vi "TPD_Controller.vi"() -> ()   [LabVIEW 2009]
uses:
  Instance           1 22Saved   TPD_Controller .vi
  <userlib>/LV-LINK/PolySubVIs/CreateAinChan.vi
  <vilib>/addons/control/pid/pid.llb/PID (DBL).vi
  <vilib>/addons/control/pid/pid.llb/PID Gain Schedule (DBL).vi
  <userlib>/LV-LINK/PolySubVIs/OLReadSingle.vi
  <vilib>/addons/control/pid/NI_PID_pid.lvlib
  <vilib>/ptbypt/NI_PtbyPt.lvlib
panel:
  out "Pyrometer Temperature [C]":dbl format="%#_4g"
  in  "OutputPower?":bool
  in  "Resistance?":bool
  out "Resistance":dbl[](array[numeric])
  out "Measured Resistance [ohms]":dbl
  out "Gain Schedule Set?":bool
  out "Temp Schedule Set?":bool
  in  "Gain Schedule":T1(array[cluster])
  in  "Gain Schedule":bool
  out "Start Sample Temperature":dbl
  out "Temperature Setpoint [C]":dbl format="%#_5g"
  in  "Thermocouple Type":string
  out "Thermocouple Temperature":dbl[](array[numeric])
  out "Thermocouple Temperature [C]":dbl
  out "Measured Voltage [V]":dbl
  out "Measured Current [A]":dbl
  in  "Set Temperature":bool
  out "Stop Running":bool
  out "Data Points":u32
  out "Pyrometer Temperature":dbl[](array[numeric])
  out "Date":string[](array[string])
  out "Time":dbl[](array[numeric])
  out "Current Setpoint":dbl[](array[numeric])
  in  "Voltage Limit [V]":dbl min=0.0 max=20.0
  in  "Temperature Limit [C]":dbl min=-273.0 max=1300.0
  in  "Current Limit [A]":dbl min=0.0 max=14.0
  in  "Save Data":bool
  in  "Notes":string
  in  "Chamber":string
  in  "Experiment Type":string
  in  "Experimenter":string
  in  "Sample":string
  in  "Stop Heating":bool
  in  "End Program":bool
  in  "Run":bool
  in  "Reset":bool
  out "Maximum Voltage":bool
  out "Voltage":dbl[](array[numeric])
  out "Current":dbl[](array[numeric])
  out "Temperature Setpoint":dbl[](array[numeric])
  out "Maximum Current":bool
  out "Temperature and Current v. Time":T2(graph)
  out "Over Voltage":bool
  out "Over Current":bool
  out "Over Temperature":bool
  out "Start Date":string
  out "Current Setpoint [A]":dbl format="%#_3g"
  in  "Temp Schedule":cluster{"time (s)":dbl, "setpoint":dbl}[](array[cluster])
  # "TPD Controller v1.1"
  # "Experiment Setup:"
  # "Hardware Setup:"
  # "Data:"
  # "Warnings:"
  # "<14A"
  # "<20V"
  # "<1300C"
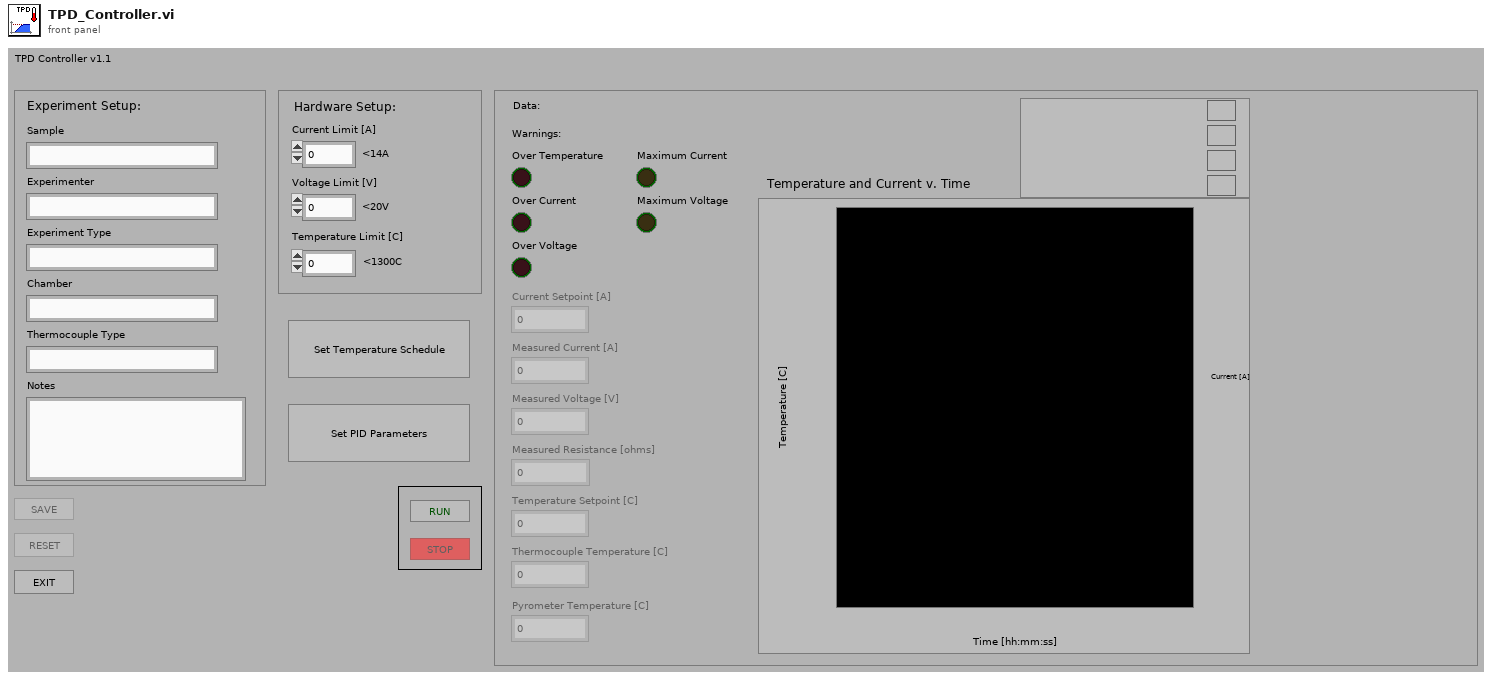
[diagram p1: front panel]
types:
  T1 = cluster{"Parameters":cluster{"Kc":dbl, "Ti":dbl, "Td":dbl}, "Maximum Temp [C]":dbl}[]
  T2 = cluster{dbl, "Temperature [C]":dbl, "setpoint":dbl, "Measured Current [A]":dbl}
  T3 = enum16{"open", "replace", "create", "open or create", "replace or create", "replace or create with confirmation"}
  T4 = cluster{"Sample":string, "Experimenter":string, "Experiment Type":string, "Chamber":string, "Thermocouple Type":string, "Notes":string}
  T5 = cluster{"proportional gain (Kc)":dbl, "integral time (Ti, min)":dbl, "derivative time (Td, min)":dbl}
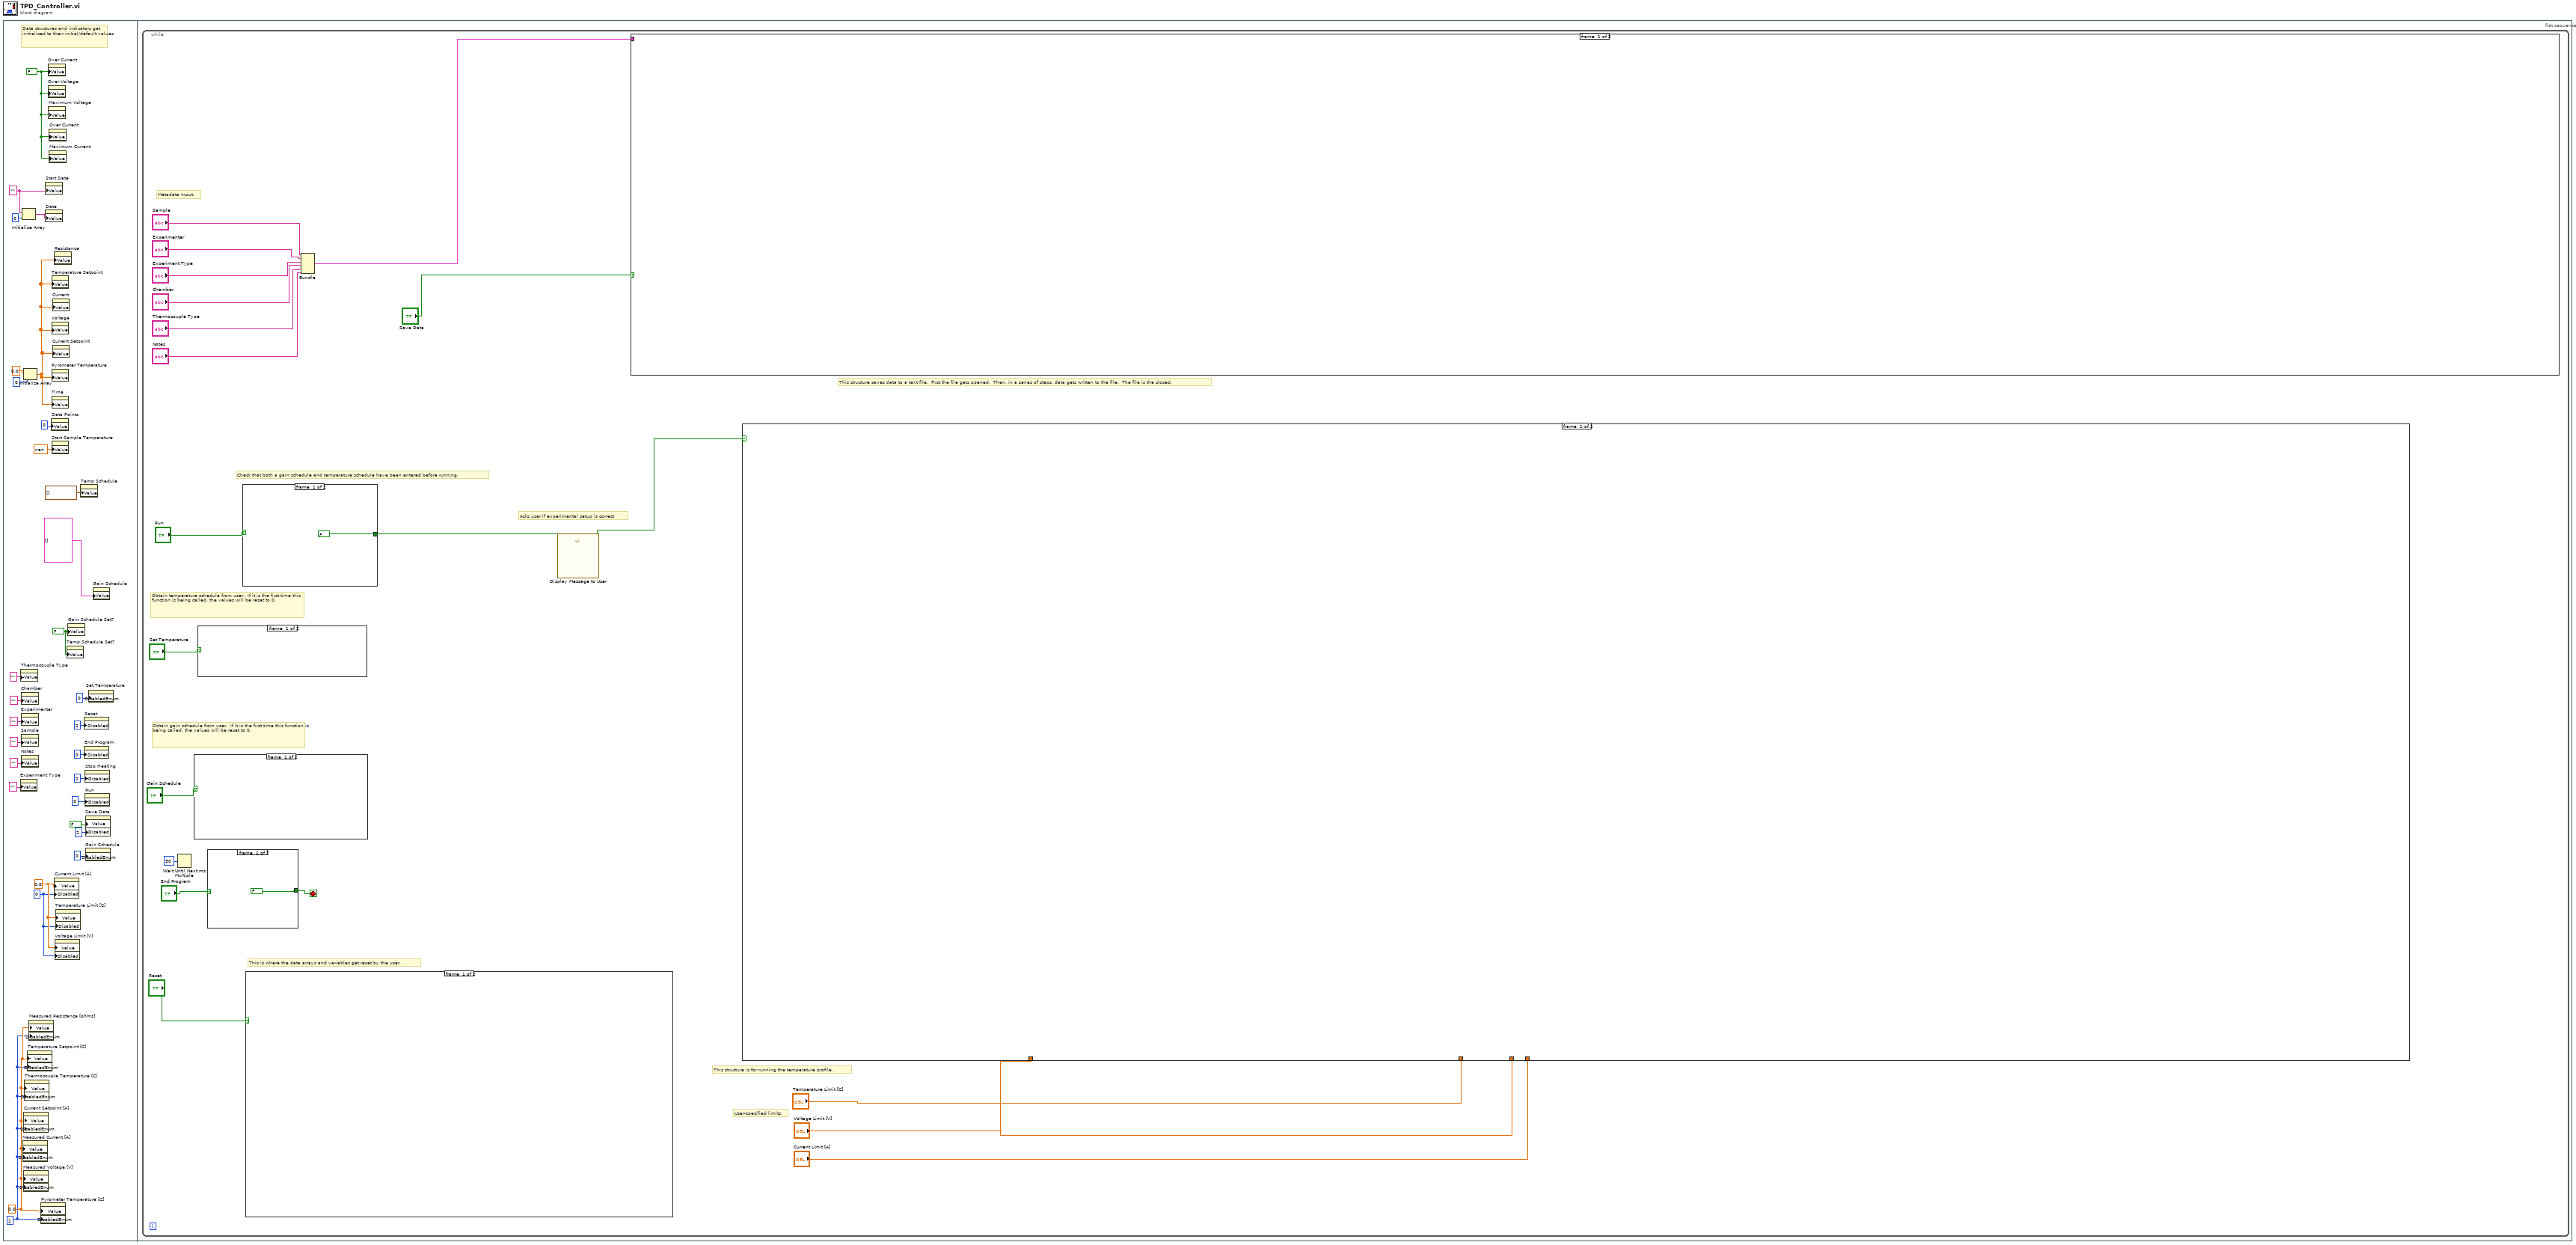
[diagram p0: block diagram]
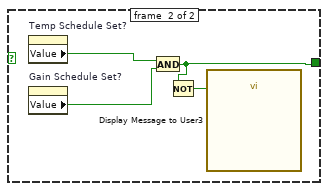
[diagram p2: hidden frame]
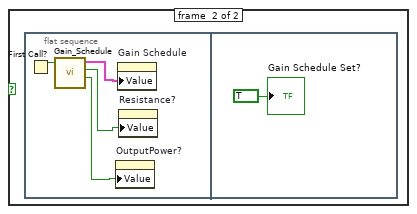
[diagram p3: hidden frame]
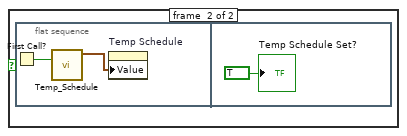
[diagram p4: hidden frame]
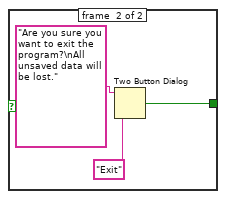
[diagram p5: hidden frame]
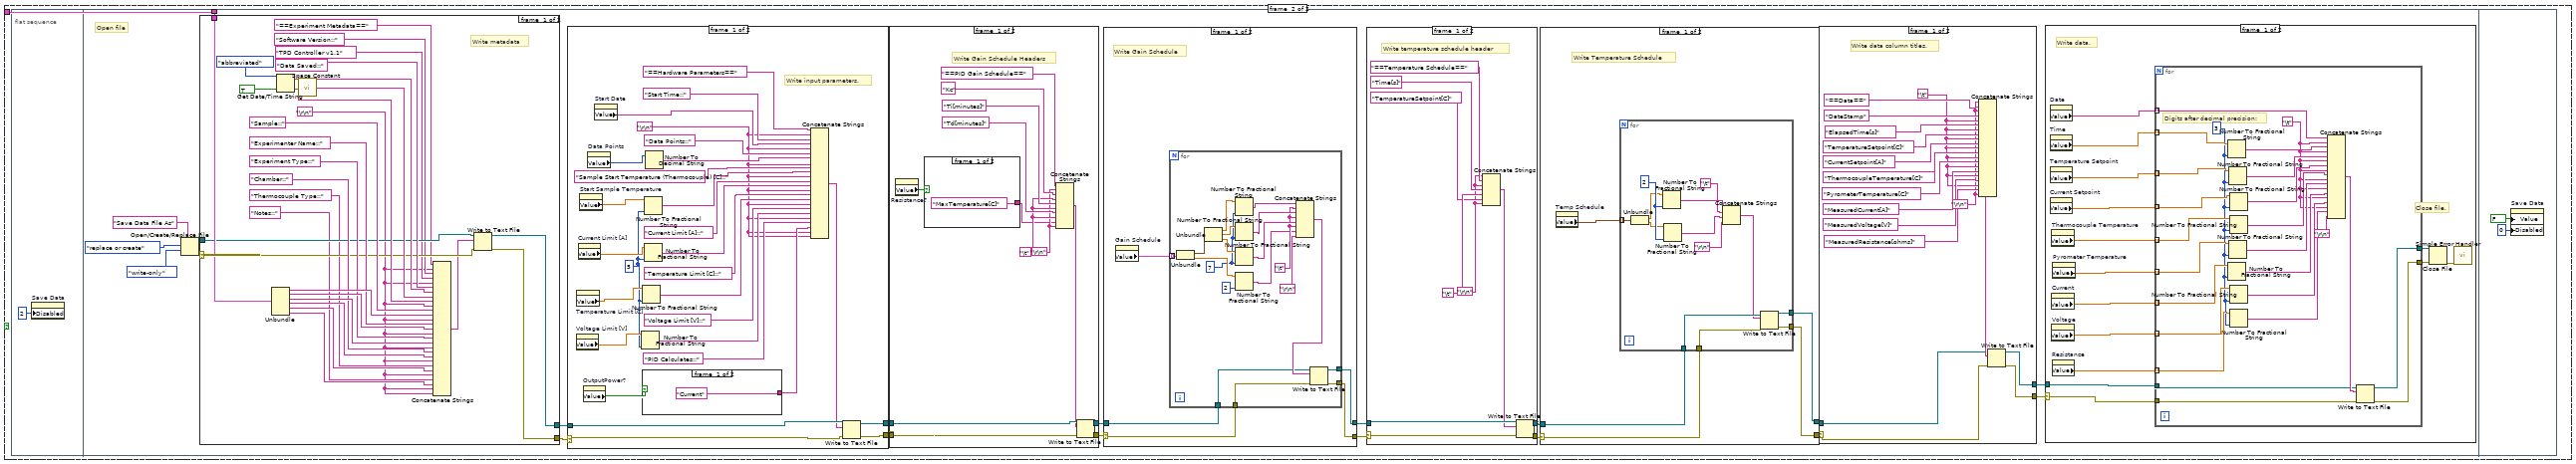
[diagram p6: hidden frame]
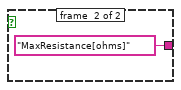
[diagram p8: hidden frame]
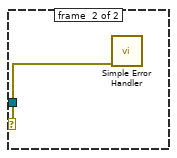
[diagram p11: hidden frame]
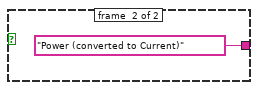
[diagram p14: hidden frame]
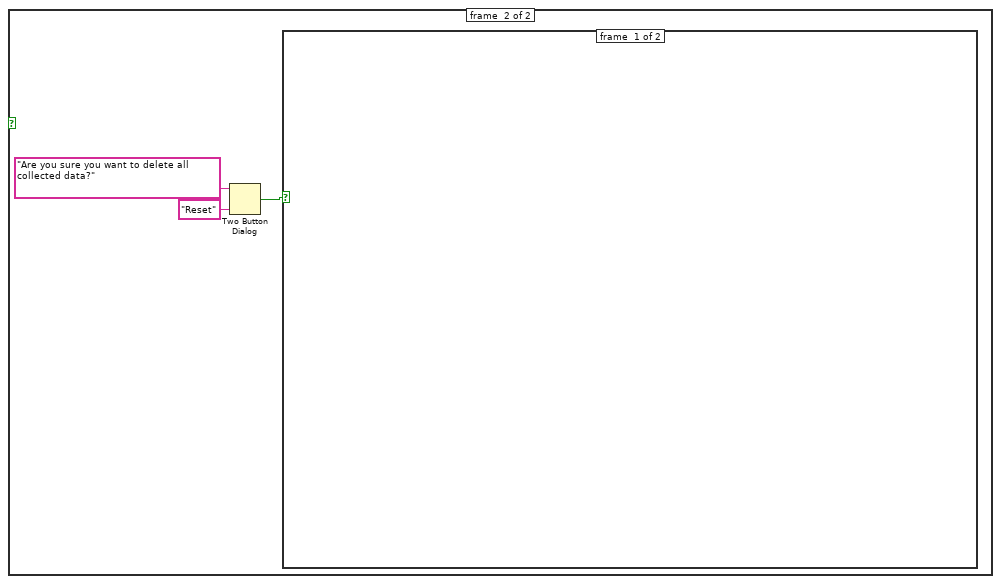
[diagram p17: hidden frame]
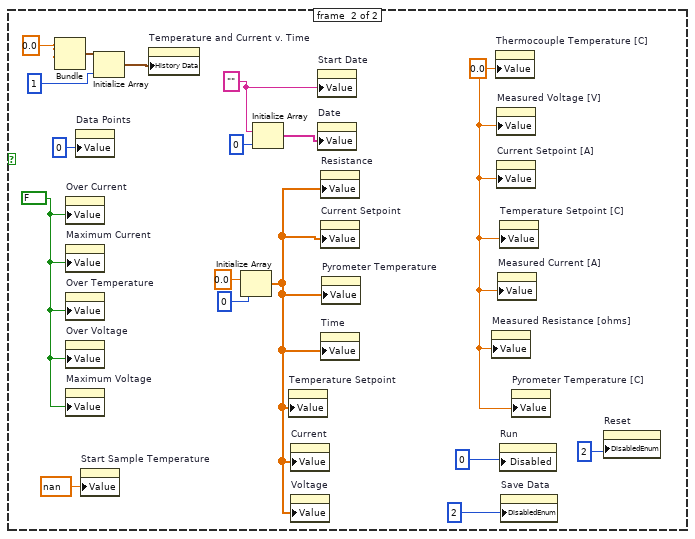
[diagram p18: hidden frame]
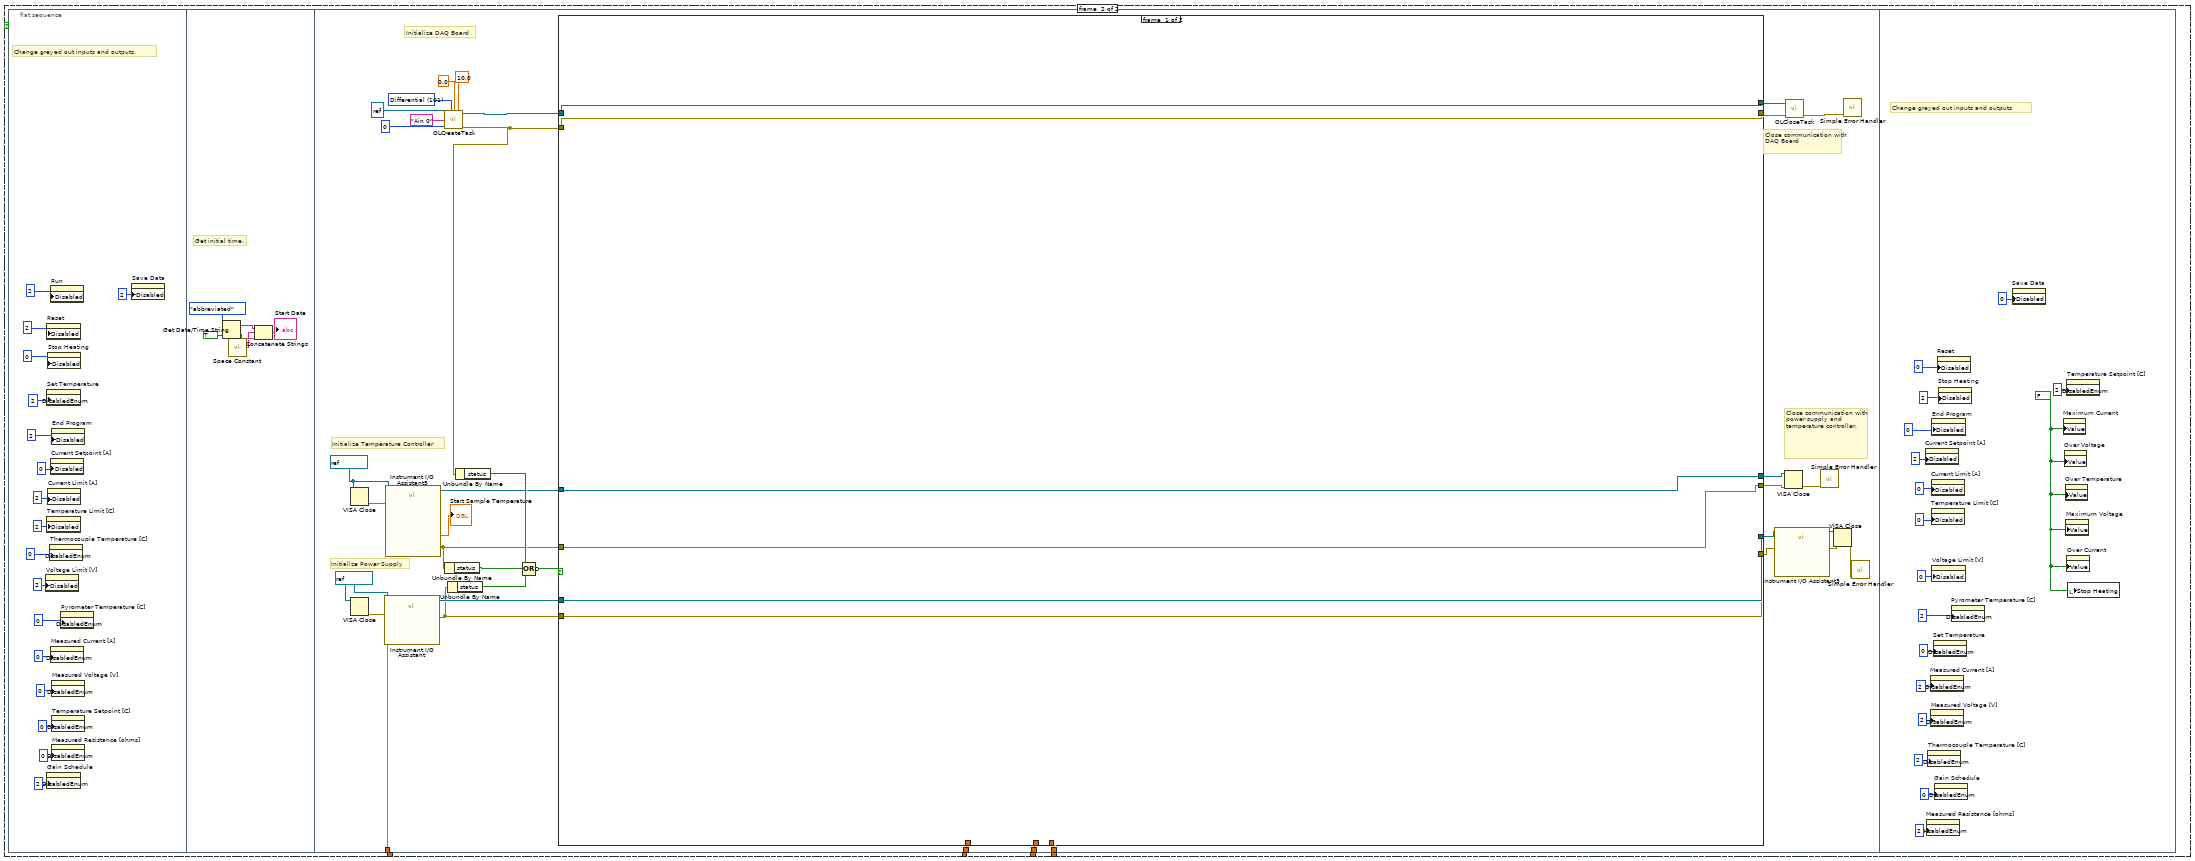
[diagram p19: hidden frame]
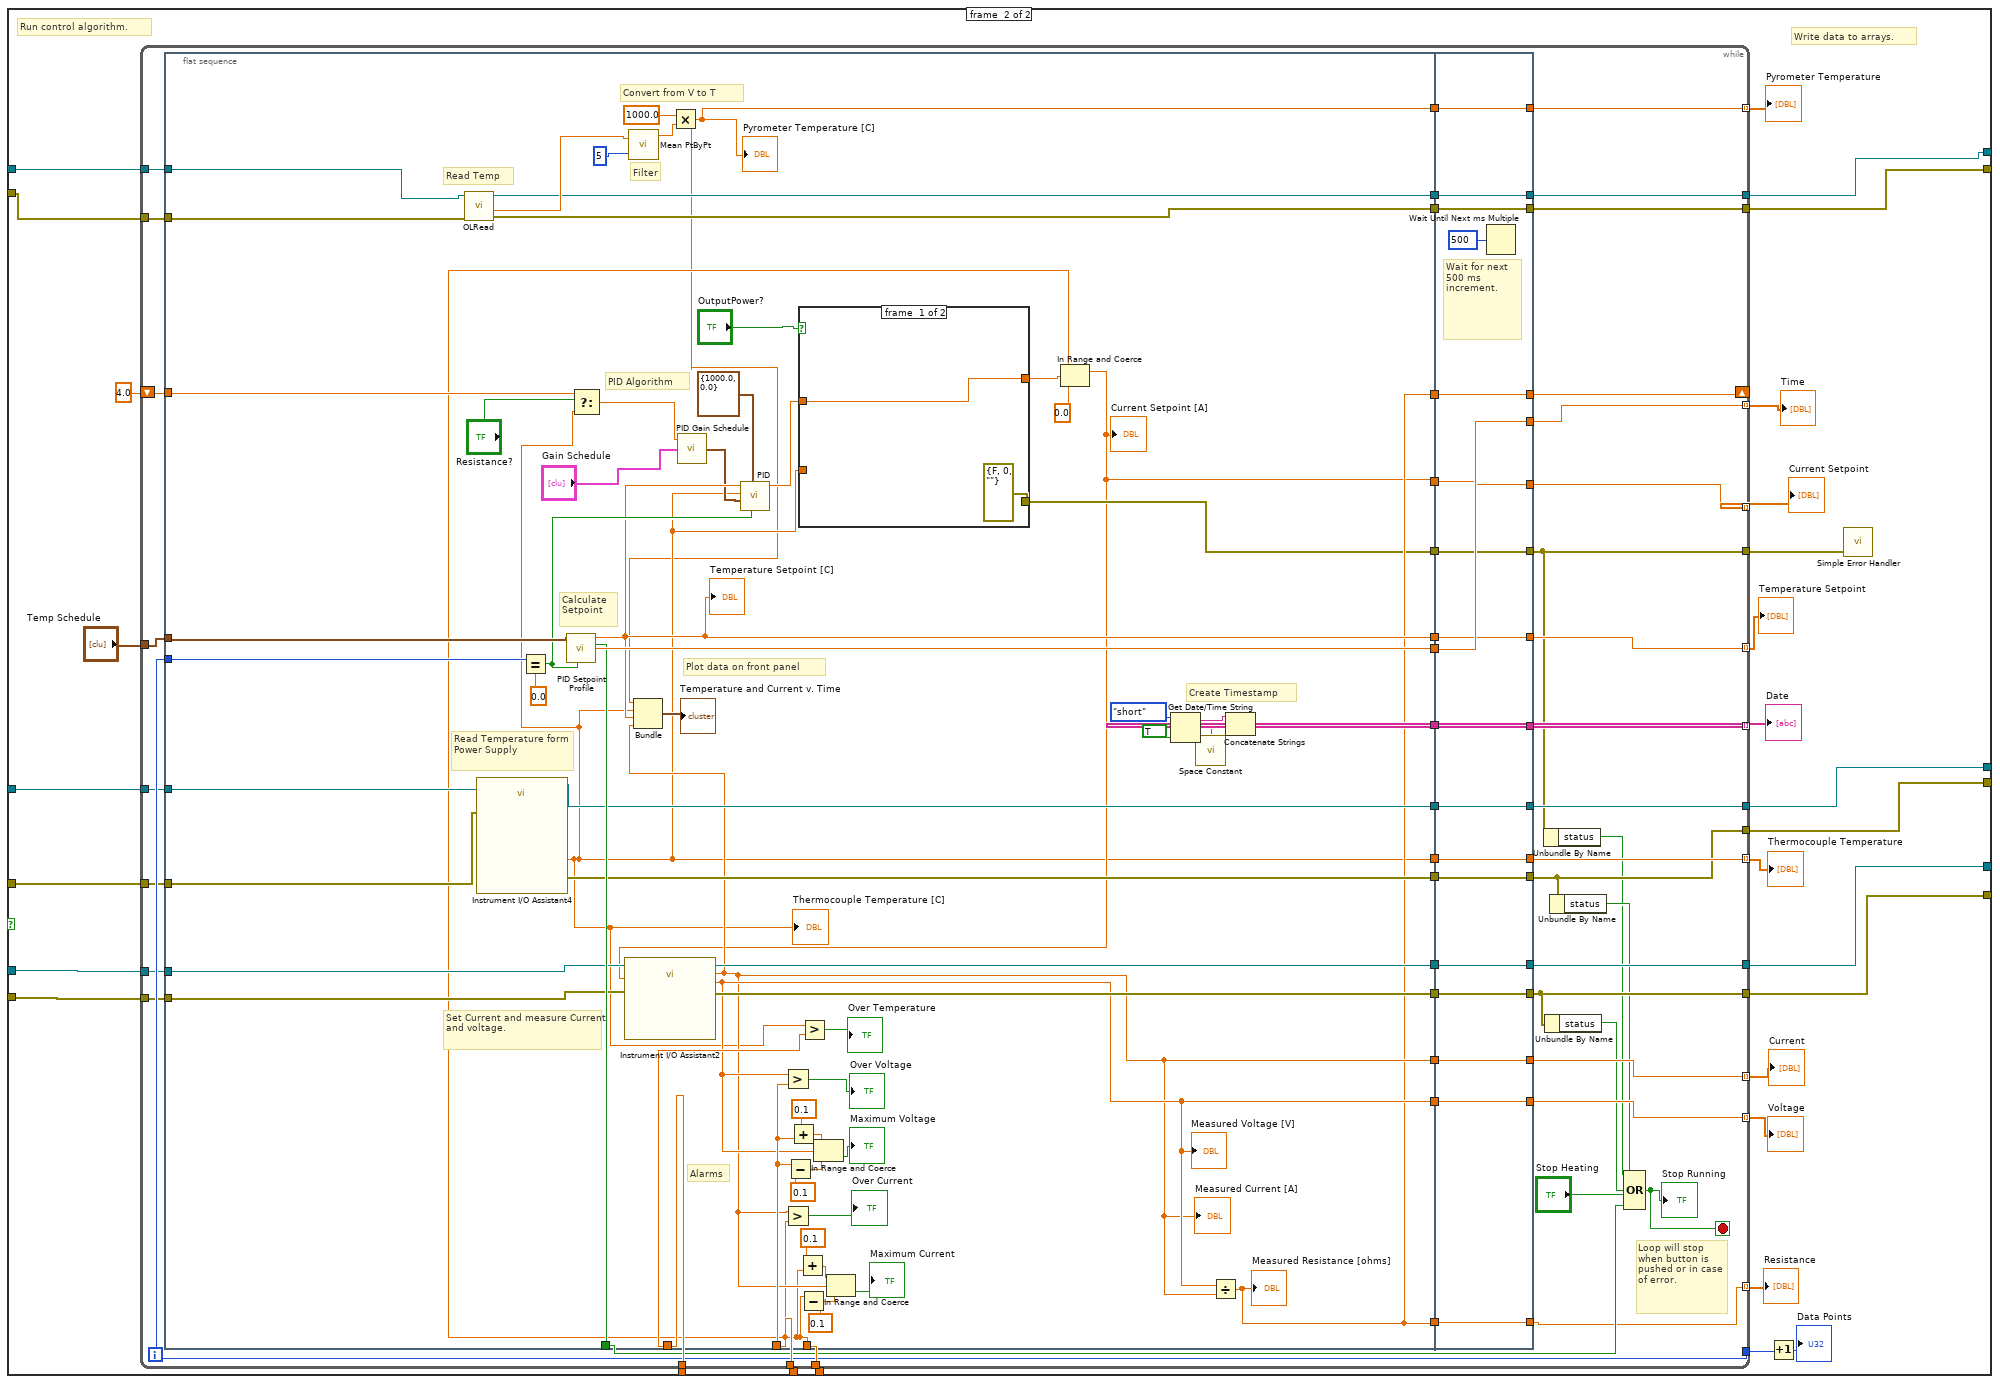
[diagram p20: hidden frame]
diagram:
  n1 = flat-sequence {
    frame #0 {
      w4 = FALSE ("Gain Schedule Set?")
      w13 = FALSE
      w11 = 0.0 ("Current Limit [A] (<11A)")
      w10 = 0
      w1 = u8 2 ("Disabled")
      w2 = 0.0 ("Current Temperature [C]")
      w23 = "" ("Start Date")
      # "Data structures and indicators get initialized to their initial/default values."
      n2 = property on="Experiment Type" class="Str"("Value"="" ("Experiment Type")) -> ()  [unwired: 2 in, 2 out]
      n3 = property on="Thermocouple Type" class="Str"("Value"="" ("Chamber")) -> ()  [unwired: 2 in, 2 out]
      n4 = property on="Chamber" class="Str"("Value"="" ("Chamber")) -> ()  [unwired: 2 in, 2 out]
      n5 = property on="Experimenter" class="Str"("Value"="" ("Experimenter")) -> ()  [unwired: 2 in, 2 out]
      n6 = property on="Sample" class="Str"("Value"="" ("Sample")) -> ()  [unwired: 2 in, 2 out]
      n7 = property on="Notes" class="Str"("Value"="" ("Notes")) -> ()  [unwired: 2 in, 2 out]
      n8 = Initialize Array(w23, 0 ("dimension size")) -> (w24:string[])
      n9 = property on="Measured Current [A]" class="DigNum (strict)"("Value"=w2, "DisabledEnum"=w1) -> ()  [unwired: 2 in, 2 out]
      n10 = Initialize Array(0.0 ("element"), 0 ("dimension size")) -> (w3:dbl[])
      n11 = property on="Measured Voltage [V]" class="DigNum (strict)"("Value"=w2, "DisabledEnum"=w1) -> ()  [unwired: 2 in, 2 out]
      n12 = property on="Current Setpoint [A]" class="DigNum (strict)"("Value"=w2, "DisabledEnum"=w1) -> ()  [unwired: 2 in, 2 out]
      n13 = property on="Thermocouple Temperature [C]" class="DigNum (strict)"("Value"=w2, "DisabledEnum"=w1) -> ()  [unwired: 2 in, 2 out]
      n14 = property on="Temperature Setpoint [C]" class="DigNum (strict)"("Value"=w2, "DisabledEnum"=w1) -> ()  [unwired: 2 in, 2 out]
      n15 = property on="Measured Resistance [ohms]" class="DigNum (strict)"("Value"=w2, "DisabledEnum"=w1) -> ()  [unwired: 2 in, 2 out]
      n16 = property on="Pyrometer Temperature [C]" class="DigNum (strict)"("Value"=w2, "DisabledEnum"=w1) -> ()  [unwired: 2 in, 2 out]
      n17 = property on="Start Date" class="Str"("Value"=w23) -> ()  [unwired: 2 in, 2 out]
      n18 = property on="Date" class="Arr (strict)"("Value"=w24) -> ()  [unwired: 2 in, 2 out]
      n19 = property on="Over Current" class="Bool (strict)"("Value"=w13) -> ()  [unwired: 2 in, 2 out]
      n20 = property on="Over Voltage" class="Bool (strict)"("Value"=w13) -> ()  [unwired: 2 in, 2 out]
      n21 = property on="Maximum Voltage" class="Bool (strict)"("Value"=w13) -> ()  [unwired: 2 in, 2 out]
      n22 = property on="Over Current" class="Bool (strict)"("Value"=w13) -> ()  [unwired: 2 in, 2 out]
      n23 = property on="Maximum Current" class="Bool (strict)"("Value"=w13) -> ()  [unwired: 2 in, 2 out]
      n24 = property on="Data Points" class="DigNum (strict)"("Value"=u32 0 ("Data Points")) -> ()  [unwired: 2 in, 2 out]
      n25 = property on="Temperature Setpoint" class="Arr (strict)"("Value"=w3) -> ()  [unwired: 2 in, 2 out]
      n26 = property on="Voltage" class="Arr (strict)"("Value"=w3) -> ()  [unwired: 2 in, 2 out]
      n27 = property on="Pyrometer Temperature" class="Arr (strict)"("Value"=w3) -> ()  [unwired: 2 in, 2 out]
      n28 = property on="Time" class="Arr (strict)"("Value"=w3) -> ()  [unwired: 2 in, 2 out]
      n29 = property on="Start Sample Temperature" class="DigNum (strict)"("Value"=nan ("Start Sample Temperature")) -> ()  [unwired: 2 in, 2 out]
      n30 = property on="Current" class="Arr (strict)"("Value"=w3) -> ()  [unwired: 2 in, 2 out]
      n31 = property on="Current Setpoint" class="Arr (strict)"("Value"=w3) -> ()  [unwired: 2 in, 2 out]
      n32 = property on="Resistance" class="Arr (strict)"("Value"=w3) -> ()  [unwired: 2 in, 2 out]
      n33 = property on="Current Limit [A]" class="DigNum (strict)"("Value"=w11, "Disabled"=w10) -> ()  [unwired: 2 in, 2 out]
      n34 = property on="Voltage Limit [V]" class="DigNum (strict)"("Value"=w11, "Disabled"=w10) -> ()  [unwired: 2 in, 2 out]
      n35 = property on="Temperature Limit [C]" class="DigNum (strict)"("Value"=w11, "Disabled"=w10) -> ()  [unwired: 2 in, 2 out]
      n36 = property on="Temp Schedule Set?" class="Bool (strict)"("Value"=w4) -> ()  [unwired: 2 in, 2 out]
      n37 = property on="Gain Schedule Set?" class="Bool (strict)"("Value"=w4) -> ()  [unwired: 2 in, 2 out]
      n38 = property on="Temp Schedule" class="Arr (strict)"("Value"=cluster{"time (s)":dbl, "setpoint":dbl}[] [] ("Temp Schedule")) -> ()  [unwired: 2 in, 2 out]
      n39 = property on="Reset" class="Bool"("Disabled"=u8 2) -> ()  [unwired: 2 in, 2 out]
      n40 = property on="End Program" class="Bool"("Disabled"=u8 0) -> ()  [unwired: 2 in, 2 out]
      n41 = property on="Stop Heating" class="Bool (strict)"("Disabled"=u8 2) -> ()  [unwired: 2 in, 2 out]
      n42 = property on="Run" class="Bool"("Disabled"=u8 0) -> ()  [unwired: 2 in, 2 out]
      n43 = property on="Save Data" class="Bool (strict)"("Value"=FALSE, "Disabled"=u8 2) -> ()  [unwired: 2 in, 2 out]
      n44 = property on="Gain Schedule" class="Bool"("DisabledEnum"=u8 0 ("Disabled")) -> ()  [unwired: 2 in, 2 out]
      n45 = property on="Set Temperature" class="Bool"("DisabledEnum"=0) -> ()  [unwired: 2 in, 2 out]
      n46 = property on="Gain Schedule" class="Arr (strict)"("Value"=T1 [] ("Gain Schedule 2")) -> ()  [unwired: 2 in, 2 out]
    }
    frame #1 {
      n47 = while {
        stop <- w42 stop-if-true
        # "Obtain gain schedule from user.  If it is the first time this function is being called, the values will be reset to 0."
        # "Check that both a gain schedule and temperature schedule have been entered before running."
        # "Obtain temperature schedule from user.  If it is the first time this function is being called, the values will be reset to 0."
        # "Asks user if experimental setup is correct"
        # "User-specified limits:"
        # "Metadata Input:"
        # "This structure saves data to a text file.  First the file gets opened.  Then, in a series of steps, data gets written to the file.  The file is the closed."
        # "This is where the data arrays and variables get reset by the user."
        # "This structure is for running the temperature profile."
        n48 = Wait Until Next ms Multiple(millisecond multiple=u32 50) -> ()  [unwired: 1 out]
        n49 = case shown="True" "Gain Schedule" {
          frame #0 {
          }
          frame #1 {
            n50 = flat-sequence {
              frame #0 {
                n51 = First Call?() -> (First Call?: T/F=w59:bool)
                n52 = call "Gain_Schedule.vi"("Initialize?"=w59) -> ("Outpower?"=w56:bool, "Resistance?"=w57:bool, "Array 2"=w58:T1)  [unwired: 8 in]
                n53 = property on="OutputPower?" class="Bool (strict)"("Value"=w56) -> ()  [unwired: 2 in, 2 out]
                n54 = property on="Gain Schedule" class="Arr (strict)"("Value"=w58) -> ()  [unwired: 2 in, 2 out]
                n55 = property on="Resistance?" class="Bool (strict)"("Value"=w57) -> ()  [unwired: 2 in, 2 out]
              }
              frame #1 {
                "Gain Schedule Set?" <- TRUE ("Gain Schedule Set?")
              }
            }
          }
        }
        n56 = case shown="True" "Set Temperature" {
          frame #0 {
          }
          frame #1 {
            n57 = flat-sequence {
              frame #0 {
                n58 = First Call?() -> (First Call?: T/F=w62:bool)
                n59 = call "Temp_Schedule.vi"("Initialize?"=w62) -> (3:w61:cluster{"time (s)":dbl, "setpoint":dbl}[])  [unwired: 9 in]
                n60 = property on="Temp Schedule" class="Arr (strict)"("Value"=w61) -> ()  [unwired: 2 in, 2 out]
              }
              frame #1 {
                "Temp Schedule Set?" <- TRUE ("Temp Schedule Set?")
              }
            }
          }
        }
        n61 = case shown="True" "End Program" {
          tunnel: [FALSE w65] -> w42
          frame #0 {
          }
          frame #1 {
            n62 = Two Button Dialog(message="Are you sure you want to exit the program?\nAll unsaved data will be lost.", 2:"Exit" ("T button name (\"OK\")")) -> (T button?=w65:bool)  [unwired: 1 in]
          }
        }
        n63 = case shown="True" "Run" {
          tunnel: [FALSE w53] -> w31
          frame #0 {
          }
          frame #1 {
            n64 = property on="Temp Schedule Set?" class="Bool (strict)"() -> ("Value"=w55:bool)  [unwired: 2 in, 2 out]
            n65 = property on="Gain Schedule Set?" class="Bool (strict)"() -> ("Value"=w54:bool)  [unwired: 2 in, 2 out]
            n66 = And(x=w55, y=w54) -> (x .and. y?=w53:bool)
            n67 = Not(x=w53) -> (.not. x?=w52:bool)
            n68 = call "Display Message to User3"("Enable"=w52) -> ()  [unwired: 9 in, 2 out]
          }
        }
        n69 = case shown="True" "Reset" {
          frame #0 {
          }
          frame #1 {
            n70 = Two Button Dialog(message="Are you sure you want to delete all collected data?", 2:"Reset" ("T button name (\"OK\")")) -> (T button?=w290:bool)  [unwired: 1 in]
            n71 = case shown="True" w290 {
              frame #0 {
              }
              frame #1 {
                w292 = 0.0 ("Thermocouple Temperature [C]")
                w298 = FALSE
                w291 = 0.0
                w307 = "" ("Start Date")
                n72 = Bundle(w291, w291, w291, w291) -> (w300:cluster{dbl, dbl, dbl, dbl})  [unwired: 1 in]
                n73 = property on="Over Current" class="Bool (strict)"("Value"=w298) -> ()  [unwired: 2 in, 2 out]
                n74 = property on="Maximum Current" class="Bool (strict)"("Value"=w298) -> ()  [unwired: 2 in, 2 out]
                n75 = property on="Over Temperature" class="Bool (strict)"("Value"=w298) -> ()  [unwired: 2 in, 2 out]
                n76 = property on="Over Voltage" class="Bool (strict)"("Value"=w298) -> ()  [unwired: 2 in, 2 out]
                n77 = property on="Maximum Voltage" class="Bool (strict)"("Value"=w298) -> ()  [unwired: 2 in, 2 out]
                n78 = property on="Data Points" class="DigNum (strict)"("Value"=u32 0 ("Data Points")) -> ()  [unwired: 2 in, 2 out]
                n79 = property on="Start Sample Temperature" class="DigNum (strict)"("Value"=nan ("Start Sample Temperature")) -> ()  [unwired: 2 in, 2 out]
                n80 = Initialize Array(w300, 1 ("dimension size")) -> (w299:cluster{dbl, dbl, dbl, dbl}[])
                n81 = property on="Temperature and Current v. Time" class="WFChart (strict)"("History Data"=w299) -> ()  [unwired: 2 in, 2 out]
                n82 = Initialize Array(0.0 ("element"), 0 ("dimension size")) -> (w295:dbl[])
                n83 = Initialize Array(w307, 0 ("dimension size")) -> (w305:string[])
                n84 = property on="Temperature Setpoint" class="Arr (strict)"("Value"=w295) -> ()  [unwired: 2 in, 2 out]
                n85 = property on="Current" class="Arr (strict)"("Value"=w295) -> ()  [unwired: 2 in, 2 out]
                n86 = property on="Voltage" class="Arr (strict)"("Value"=w295) -> ()  [unwired: 2 in, 2 out]
                n87 = property on="Start Date" class="Str"("Value"=w307) -> ()  [unwired: 2 in, 2 out]
                n88 = property on="Date" class="Arr (strict)"("Value"=w305) -> ()  [unwired: 2 in, 2 out]
                n89 = property on="Resistance" class="Arr (strict)"("Value"=w295) -> ()  [unwired: 2 in, 2 out]
                n90 = property on="Current Setpoint" class="Arr (strict)"("Value"=w295) -> ()  [unwired: 2 in, 2 out]
                n91 = property on="Time" class="Arr (strict)"("Value"=w295) -> ()  [unwired: 2 in, 2 out]
                n92 = property on="Pyrometer Temperature" class="Arr (strict)"("Value"=w295) -> ()  [unwired: 2 in, 2 out]
                n93 = property on="Measured Resistance [ohms]" class="DigNum (strict)"("Value"=w292) -> ()  [unwired: 2 in, 2 out]
                n94 = property on="Thermocouple Temperature [C]" class="DigNum (strict)"("Value"=w292) -> ()  [unwired: 2 in, 2 out]
                n95 = property on="Measured Voltage [V]" class="DigNum (strict)"("Value"=w292) -> ()  [unwired: 2 in, 2 out]
                n96 = property on="Current Setpoint [A]" class="DigNum (strict)"("Value"=w292) -> ()  [unwired: 2 in, 2 out]
                n97 = property on="Measured Current [A]" class="DigNum (strict)"("Value"=w292) -> ()  [unwired: 2 in, 2 out]
                n98 = property on="Temperature Setpoint [C]" class="DigNum (strict)"("Value"=w292) -> ()  [unwired: 2 in, 2 out]
                n99 = property on="Run" class="Bool"("Disabled"=0) -> ()  [unwired: 2 in, 2 out]
                n100 = property on="Save Data" class="Bool (strict)"("DisabledEnum"=2 ("Disabled")) -> ()  [unwired: 2 in, 2 out]
                n101 = property on="Pyrometer Temperature [C]" class="DigNum (strict)"("Value"=w292) -> ()  [unwired: 2 in, 2 out]
                n102 = property on="Reset" class="Bool"("DisabledEnum"=2 ("Disabled")) -> ()  [unwired: 2 in, 2 out]
              }
            }
          }
        }
        n103 = Bundle("Sample"="Sample", "Experimenter"="Experimenter", "Experiment Type"="Experiment Type", "Chamber"="Chamber", "Thermocouple Type"="Thermocouple Type", "Notes"="Notes") -> (w44:T4)  [unwired: 1 in]
        n104 = call "Display Message to User"("Enable"=w31) -> ("Yes"=w39:bool)  [unwired: 9 in, 1 out]
        n105 = case shown="True" "Save Data" {
          tunnel: w44 -> [_ w68]
          frame #0 {
          }
          frame #1 {
            n106 = flat-sequence {
              tunnel: w68 -> [w85]
              frame #0 {
                n107 = property on="Save Data" class="Bool (strict)"("Disabled"=u8 2) -> ()  [unwired: 2 in, 2 out]
              }
              frame #1 {
                # "Open file"
                n108 = Open/Create/Replace File(prompt="Save Data File As", operation (0:open)=T3."replace or create", access (0:read/write)=enum16{"read/write", "read-only", "write-only"}."write-only") -> (refnum out=w84:refnum<file>, error out=w86:errorcluster)  [unwired: 3 in, 1 out]
                n109 = case shown="No Error" w86 {
                  selector: w86 -> [w269 w285]
                  tunnel: w85 -> [w283 _]
                  tunnel: w84 -> [w267 w284]
                  tunnel: [w266 w285] -> w83
                  tunnel: [w265 w284] -> w82
                  frame #0 {
                    w256 = "\r\n"
                    # "Write metadata"
                    n110 = Unbundle(w283) -> ("Sample"=w277:string, "Experimenter"=w275:string, "Experiment Type"=w273:string, "Chamber"=w271:string, "Thermocouple Type"=w270:string, "Notes"=w258:string)
                    n111 = Get Date/Time String(date format (0)=enum16{"short", "long", "abbreviated"}."abbreviated", want seconds? (F)=TRUE) -> (date string=w281:string, time string=w279:string)  [unwired: 1 in]
                    n112 = call <vilib>:"Space Constant.vi"() -> ("String"=w280:string)
                    n113 = Concatenate Strings("==Experiment Metadata==", w256, "Software Version::", "TPD Controller v1.1", w256, "Data Saved::", w281, w280, w279, w256, "Sample::", w277, w256, "Experimenter Name::", w275, w256, "Experiment Type::", w273, w256, "Chamber::", w271, w256, "Thermocouple Type::", w270, w256, "Notes::", w258, w256, w256) -> (w268:string)
                    n114 = Write to Text File(file (use dialog)=w267, text=w268, error in=w269) -> (refnum out=w265:refnum<file>, error out=w266:errorcluster)  [unwired: 1 in, 1 out]
                  }
                  frame #1 {
                  }
                }
                n115 = case shown="No Error" w83 {
                  selector: w83 -> [w243 w255]
                  tunnel: w82 -> [w244 w254]
                  tunnel: [w238 w255] -> w74
                  tunnel: [w237 w254] -> w75
                  frame #0 {
                    w229 = i16 5 ("precision (6)")
                    w224 = "\r\n"
                    # "Write input parameters."
                    n116 = property on="Voltage Limit [V]" class="DigNum (strict)"() -> ("Value"=w239:dbl)  [unwired: 2 in, 2 out]
                    n117 = property on="Temperature Limit [C]" class="DigNum (strict)"() -> ("Value"=w240:dbl)  [unwired: 2 in, 2 out]
                    n118 = property on="Current Limit [A]" class="DigNum (strict)"() -> ("Value"=w241:dbl)  [unwired: 2 in, 2 out]
                    n119 = property on="Start Sample Temperature" class="DigNum (strict)"() -> ("Value"=w232:dbl)  [unwired: 2 in, 2 out]
                    n120 = property on="OutputPower?" class="Bool (strict)"() -> ("Value"=w226:bool)  [unwired: 2 in, 2 out]
                    n121 = property on="Data Points" class="DigNum (strict)"() -> ("Value"=w235:u32)  [unwired: 2 in, 2 out]
                    n122 = property on="Start Date" class="Str"() -> ("Value"=w236:string)  [unwired: 2 in, 2 out]
                    n123 = Number To Fractional String(number=w239, precision (6)=w229) -> (F-format string=w233:string)  [unwired: 2 in]
                    n124 = Number To Fractional String(number=w240, precision (6)=w229) -> (F-format string=w245:string)  [unwired: 2 in]
                    n125 = case shown="True" w226 {
                      tunnel: ["Current" "Power (converted to Current)"] -> w225
                      frame #0 {
                      }
                      frame #1 {
                      }
                    }
                    n126 = Number To Fractional String(number=w232, precision (6)=w229) -> (F-format string=w231:string)  [unwired: 2 in]
                    n127 = Number To Fractional String(number=w241, precision (6)=w229) -> (F-format string=w247:string)  [unwired: 2 in]
                    n128 = Number To Decimal String(number=w235) -> (decimal integer string=w249:string)  [unwired: 1 in]
                    n129 = Concatenate Strings("==Hardware Parameters==", w224, "Start Time::", w236, w224, "Data Points::", w249, w224, "Sample Start Temperature (Thermocouple) [C]::", w231, w224, "Current Limit [A]::", w247, w224, "Temperature Limit [C]::", w245, w224, "Voltage Limit [V]::", w233, w224, "PID Calculates::", w225, w224, w224) -> (w242:string)
                    n130 = Write to Text File(file (use dialog)=w244, text=w242, error in=w243) -> (refnum out=w237:refnum<file>, error out=w238:errorcluster)  [unwired: 1 in, 1 out]
                  }
                  frame #1 {
                  }
                }
                n131 = case shown="No Error" w74 {
                  selector: w74 -> [w125 w131]
                  tunnel: w74 -> [_ _]
                  tunnel: [w127 w132] -> w72
                  tunnel: w75 -> [w126 w132]
                  tunnel: [w128 w131] -> w73
                  frame #0 {
                    w120 = "\t"
                    w119 = "\r\n"
                    # "Write Gain Schedule Headers"
                    n132 = property on="Resistance?" class="Bool (strict)"() -> ("Value"=w117:bool)  [unwired: 2 in, 2 out]
                    n133 = case shown="True" w117 {
                      tunnel: ["MaxTemperature[C]" "MaxResistance[ohms]"] -> w116
                      frame #0 {
                      }
                      frame #1 {
                      }
                    }
                    n134 = Concatenate Strings("==PID Gain Schedule==", w119, "Kc", w120, "Ti[minutes]", w120, "Td[minutes]", w120, w116, w119) -> (w118:string)
                    n135 = Write to Text File(file (use dialog)=w126, text=w118, error in=w125) -> (refnum out=w127:refnum<file>, error out=w128:errorcluster)  [unwired: 1 in, 1 out]
                  }
                  frame #1 {
                  }
                }
                n136 = case shown="No Error" w73 {
                  selector: w73 -> [w92 w114]
                  tunnel: w72 -> [w93 w115]
                  tunnel: [w91 w115] -> w71
                  tunnel: [w90 w114] -> w70
                  frame #0 {
                    # "Write Gain Schedule"
                    n137 = property on="Gain Schedule" class="Arr (strict)"() -> ("Value"=w94:T1)  [unwired: 2 in, 2 out]
                    n138 = for {
                      tunnel: w94 -> [w113] mode=indexing
                      tunnel: w93 -> [w98]
                      tunnel: w92 -> [w97]
                      tunnel: [w96] -> w90
                      tunnel: [w95] -> w91
                      w107 = i16 7 ("precision (6)")
                      w102 = "\t"
                      n139 = Unbundle(w113) -> ("Parameters"=w112:cluster{"Kc":dbl, "Ti":dbl, "Td":dbl}, "Maximum Temp [C]"=w108:dbl)
                      n140 = Unbundle(w112) -> ("Kc"=w111:dbl, "Ti"=w110:dbl, "Td"=w109:dbl)
                      n141 = Number To Fractional String(number=w111, precision (6)=w107) -> (F-format string=w105:string)  [unwired: 2 in]
                      n142 = Number To Fractional String(number=w110, precision (6)=w107) -> (F-format string=w104:string)  [unwired: 2 in]
                      n143 = Number To Fractional String(number=w109, precision (6)=w107) -> (F-format string=w103:string)  [unwired: 2 in]
                      n144 = Number To Fractional String(number=w108, precision (6)=i16 2) -> (F-format string=w101:string)  [unwired: 2 in]
                      n145 = Concatenate Strings(w105, w102, w104, w102, w103, w102, w101, "\r\n") -> (w99:string)
                      n146 = Write to Text File(file (use dialog)=w98, text=w99, error in=w97) -> (refnum out=w95:refnum<file>, error out=w96:errorcluster)  [unwired: 1 in, 1 out]
                    }
                  }
                  frame #1 {
                  }
                }
                n147 = case shown="No Error" w70 {
                  selector: w70 -> [w200 w203]
                  tunnel: w71 -> [w199 w204]
                  tunnel: [w202 w204] -> w78
                  tunnel: [w201 w203] -> w79
                  frame #0 {
                    w193 = "\r\n"
                    # "Write temperature schedule header"
                    n148 = Concatenate Strings(w193, "==Temperature Schedule==", w193, "Time[s]", "\t", "TemperatureSetpoint[C]", w193) -> (w195:string)
                    n149 = Write to Text File(file (use dialog)=w199, text=w195, error in=w200) -> (refnum out=w202:refnum<file>, error out=w201:errorcluster)  [unwired: 1 in, 1 out]
                  }
                  frame #1 {
                  }
                }
                n150 = case shown="No Error" w79 {
                  selector: w79 -> [w133 w151]
                  tunnel: w78 -> [w134 w152]
                  tunnel: [w137 w152] -> w77
                  tunnel: [w136 w151] -> w76
                  frame #0 {
                    # "Write Temperature Schedule"
                    n151 = property on="Temp Schedule" class="Arr (strict)"() -> ("Value"=w135:cluster{"time (s)":dbl, "setpoint":dbl}[])  [unwired: 2 in, 2 out]
                    n152 = for {
                      tunnel: [w150] -> w137
                      tunnel: [w149] -> w136
                      tunnel: w135 -> [w148] mode=indexing
                      tunnel: w134 -> [w140]
                      tunnel: w133 -> [w139]
                      w147 = i16 2 ("precision (6)")
                      n153 = Unbundle(w148) -> ("time (s)"=w146:dbl, "setpoint"=w145:dbl)
                      n154 = Number To Fractional String(number=w146, precision (6)=w147) -> (F-format string=w144:string)  [unwired: 2 in]
                      n155 = Number To Fractional String(number=w145, precision (6)=w147) -> (F-format string=w142:string)  [unwired: 2 in]
                      n156 = Concatenate Strings(w144, "\t", w142, "\r\n") -> (w138:string)
                      n157 = Write to Text File(file (use dialog)=w140, text=w138, error in=w139) -> (refnum out=w150:refnum<file>, error out=w149:errorcluster)  [unwired: 1 in, 1 out]
                    }
                  }
                  frame #1 {
                  }
                }
                n158 = case shown="No Error" w76 {
                  selector: w76 -> [w215 w222]
                  tunnel: w77 -> [w209 w223]
                  tunnel: [w214 w223] -> w81
                  tunnel: [w213 w222] -> w80
                  frame #0 {
                    w205 = "\r\n"
                    w207 = "\t"
                    # "Write data column titles."
                    n159 = Concatenate Strings(w205, "==Data==", w205, "DateStamp", w207, "ElapsedTime[s]", w207, "TemperatureSetpoint[C]", w207, "CurrentSetpoint[A]", w207, "ThermocoupleTemperature[C]", w207, "PyrometerTemperature[C]", w207, "MeasuredCurrent[A]", w207, "MeasuredVoltage[V]", w207, "MeasuredResistance[ohms]", w205) -> (w216:string)
                    n160 = Write to Text File(file (use dialog)=w209, text=w216, error in=w215) -> (refnum out=w214:refnum<file>, error out=w213:errorcluster)  [unwired: 1 in, 1 out]
                  }
                  frame #1 {
                  }
                }
                n161 = case shown="No Error" w80 {
                  selector: w80 -> [w165 w192]
                  tunnel: w81 -> [w166 _]
                  frame #0 {
                    # "Close file."
                    # "Write data."
                    n162 = property on="Date" class="Arr (strict)"() -> ("Value"=w162:string[])  [unwired: 2 in, 2 out]
                    n163 = property on="Time" class="Arr (strict)"() -> ("Value"=w161:dbl[])  [unwired: 2 in, 2 out]
                    n164 = property on="Temperature Setpoint" class="Arr (strict)"() -> ("Value"=w159:dbl[])  [unwired: 2 in, 2 out]
                    n165 = property on="Current Setpoint" class="Arr (strict)"() -> ("Value"=w160:dbl[])  [unwired: 2 in, 2 out]
                    n166 = property on="Thermocouple Temperature" class="Arr (strict)"() -> ("Value"=w154:dbl[])  [unwired: 2 in, 2 out]
                    n167 = property on="Current" class="Arr (strict)"() -> ("Value"=w157:dbl[])  [unwired: 2 in, 2 out]
                    n168 = property on="Voltage" class="Arr (strict)"() -> ("Value"=w156:dbl[])  [unwired: 2 in, 2 out]
                    n169 = property on="Resistance" class="Arr (strict)"() -> ("Value"=w153:dbl[])  [unwired: 2 in, 2 out]
                    n170 = property on="Pyrometer Temperature" class="Arr (strict)"() -> ("Value"=w158:dbl[])  [unwired: 2 in, 2 out]
                    n171 = for {
                      tunnel: w162 -> [w191] mode=indexing
                      tunnel: w161 -> [w189] mode=indexing
                      tunnel: w166 -> [w185]
                      tunnel: w165 -> [w184]
                      tunnel: [w183] -> w164
                      tunnel: [w182] -> w163
                      tunnel: w159 -> [w181] mode=indexing
                      tunnel: w160 -> [w180] mode=indexing
                      tunnel: w158 -> [w175] mode=indexing
                      tunnel: w157 -> [w174] mode=indexing
                      tunnel: w156 -> [w173] mode=indexing
                      tunnel: w154 -> [w176] mode=indexing
                      tunnel: w153 -> [w171] mode=indexing
                      w170 = i16 3 ("precision (6)")
                      w169 = "\t"
                      # "Digits after decimal precision:"
                      n172 = Number To Fractional String(number=w174, precision (6)=w170) -> (F-format string=w177:string)  [unwired: 2 in]
                      n173 = Number To Fractional String(number=w189, precision (6)=w170) -> (F-format string=w190:string)  [unwired: 2 in]
                      n174 = Number To Fractional String(number=w181, precision (6)=w170) -> (F-format string=w188:string)  [unwired: 2 in]
                      n175 = Number To Fractional String(number=w175, precision (6)=w170) -> (F-format string=w178:string)  [unwired: 2 in]
                      n176 = Number To Fractional String(number=w176, precision (6)=w170) -> (F-format string=w179:string)  [unwired: 2 in]
                      n177 = Number To Fractional String(number=w173, precision (6)=w170) -> (F-format string=w172:string)  [unwired: 2 in]
                      n178 = Number To Fractional String(number=w171, precision (6)=w170) -> (F-format string=w168:string)  [unwired: 2 in]
                      n179 = Number To Fractional String(number=w180, precision (6)=w170) -> (F-format string=w187:string)  [unwired: 2 in]
                      n180 = Concatenate Strings(w191, w169, w190, w169, w188, w169, w187, w169, w179, w169, w178, w169, w177, w169, w172, w169, w168, "\r\n") -> (w186:string)
                      n181 = Write to Text File(file (use dialog)=w185, text=w186, error in=w184) -> (refnum out=w183:refnum<file>, error out=w182:errorcluster)  [unwired: 1 in, 1 out]
                    }
                    n182 = Close File(refnum=w164, error in=w163) -> (error out=w155:errorcluster)  [unwired: 1 out]
                    n183 = call <vilib>:"Simple Error Handler.vi"("error in (no error)"=w155) -> ()  [unwired: 4 in, 5 out]
                  }
                  frame #1 {
                    n184 = call <vilib>:"Simple Error Handler.vi"("error in (no error)"=w192) -> ()  [unwired: 4 in, 5 out]
                  }
                }
              }
              frame #2 {
                n185 = property on="Save Data" class="Bool (strict)"("Value"=FALSE ("Save Data"), "Disabled"=u8 0) -> ()  [unwired: 2 in, 2 out]
              }
            }
          }
        }
        n186 = case shown="True" w39 {
          tunnel: "Current Limit [A]" -> [_ w311]
          tunnel: "Voltage Limit [V]" -> [_ w310]
          tunnel: "Temperature Limit [C]" -> [_ w309]
          tunnel: "Voltage Limit [V]" -> [_ w308]
          frame #0 {
          }
          frame #1 {
            n187 = flat-sequence {
              tunnel: w311 -> [w370]
              tunnel: w310 -> [w369]
              tunnel: w309 -> [w368]
              tunnel: w308 -> [w361]
              frame #0 {
                # "Change greyed out inputs and outputs."
                n188 = property on="Voltage Limit [V]" class="DigNum (strict)"("Disabled"=2) -> ()  [unwired: 2 in, 2 out]
                n189 = property on="Reset" class="Bool"("Disabled"=2) -> ()  [unwired: 2 in, 2 out]
                n190 = property on="Set Temperature" class="Bool"("DisabledEnum"=2) -> ()  [unwired: 2 in, 2 out]
                n191 = property on="Temperature Limit [C]" class="DigNum (strict)"("Disabled"=2) -> ()  [unwired: 2 in, 2 out]
                n192 = property on="Gain Schedule" class="Bool"("DisabledEnum"=2) -> ()  [unwired: 2 in, 2 out]
                n193 = property on="Stop Heating" class="Bool (strict)"("Disabled"=0) -> ()  [unwired: 2 in, 2 out]
                n194 = property on="Current Limit [A]" class="DigNum (strict)"("Disabled"=2) -> ()  [unwired: 2 in, 2 out]
                n195 = property on="Thermocouple Temperature [C]" class="DigNum (strict)"("DisabledEnum"=0) -> ()  [unwired: 2 in, 2 out]
                n196 = property on="Run" class="Bool"("Disabled"=2) -> ()  [unwired: 2 in, 2 out]
                n197 = property on="Current Setpoint [A]" class="DigNum (strict)"("Disabled"=u8 0) -> ()  [unwired: 2 in, 2 out]
                n198 = property on="Measured Current [A]" class="DigNum (strict)"("DisabledEnum"=0) -> ()  [unwired: 2 in, 2 out]
                n199 = property on="End Program" class="Bool"("Disabled"=2) -> ()  [unwired: 2 in, 2 out]
                n200 = property on="Measured Voltage [V]" class="DigNum (strict)"("DisabledEnum"=0) -> ()  [unwired: 2 in, 2 out]
                n201 = property on="Temperature Setpoint [C]" class="DigNum (strict)"("DisabledEnum"=0) -> ()  [unwired: 2 in, 2 out]
                n202 = property on="Measured Resistance [ohms]" class="DigNum (strict)"("DisabledEnum"=0) -> ()  [unwired: 2 in, 2 out]
                n203 = property on="Pyrometer Temperature [C]" class="DigNum (strict)"("DisabledEnum"=u8 0 ("Disabled")) -> ()  [unwired: 2 in, 2 out]
                n204 = property on="Save Data" class="Bool (strict)"("Disabled"=u8 2) -> ()  [unwired: 2 in, 2 out]
              }
              frame #1 {
                # "Get initial time."
                n205 = Get Date/Time String(date format (0)=enum16{"short", "long", "abbreviated"}."abbreviated", want seconds? (F)=TRUE) -> (date string=w331:string, time string=w330:string)  [unwired: 1 in]
                n206 = call <vilib>:"Space Constant.vi"() -> ("String"=w329:string)
                n207 = Concatenate Strings(w331, w329, w330) -> (→"Start Date":string)
              }
              frame #2 {
                w345 = refnum<visa-resource-name> "COM8" ("VISA resource name")
                w347 = refnum<visa-resource-name> "COM1" ("VISA resource name")
                w367 = 101 items=["SingleEnded"=100, "Differential"=101] ("Channel Type")
                # "Close communication with power supply and temperature controller."
                # "Initialize Power Supply"
                # "Initialize Temperature Controller"
                # "Close communication with DAQ Board"
                # "Initialize DAQ Board"
                n208 = VISA Close(VISA resource name=w345) -> (error out=w346:errorcluster)  [unwired: 1 in]
                n209 = VISA Close(VISA resource name=w347) -> (error out=w348:errorcluster)  [unwired: 1 in]
                n210 = call "Instrument I/O Assistant"("Session In"=w345, "Max Voltage [V]"=w361, "error in"=w346) -> ("Session Out"=w360:refnum<visa-resource-name>, "error out"=w359:errorcluster)  [unwired: 23 in]
                n211 = call "Instrument I/O Assistant5"("Session In"=w347, "error in"=w348) -> ("Session Out"=w350:refnum<visa-resource-name>, "Temperature [C]"=→"Start Sample Temperature":dbl, "error out"=w349:errorcluster)  [unwired: 23 in]
                n212 = call-poly <userlib>:"OLCreateTask.vi"("Task In"=refnum<k24> refnum, "Channel Type"=w367, "Range Min"=0.0, "Range Max"=10.0, "Channel"="Ain 0", "Element"=0) -> ("Task Out"=w344:refnum<k24>, "error out"=w343:errorcluster)  [unwired: 8 in]
                n213 = Unbundle By Name(w349) -> ("status"=w353:bool)
                n214 = Unbundle By Name(w359) -> ("status"=w362:bool)
                n215 = Unbundle By Name(w343) -> ("status"=w352:bool)
                n216 = Compound Arithmetic op=OR(w352, w353, w362) -> (invert w363:bool)
                n217 = case shown="True" w363 {
                  tunnel: w370 -> [_ w405]
                  tunnel: w369 -> [_ w404]
                  tunnel: w368 -> [_ w403]
                  tunnel: w343 -> [w376 w382]
                  tunnel: w344 -> [w375 w383]
                  tunnel: [w375 w381] -> w341
                  tunnel: [w376 w380] -> w342
                  tunnel: w360 -> [w374 w393]
                  tunnel: w359 -> [w373 w392]
                  tunnel: [w374 w391] -> w358
                  tunnel: [w373 w390] -> w357
                  tunnel: w350 -> [w372 w388]
                  tunnel: w349 -> [w371 w387]
                  tunnel: [w372 w378] -> w336
                  tunnel: [w371 w377] -> w335
                  frame #0 {
                  }
                  frame #1 {
                    # "Write data to arrays."
                    # "Run control algorithm."
                    n218 = while {
                      tunnel: [w454] -> w402 mode=indexing
                      tunnel: [w457] -> w401 mode=indexing
                      tunnel: [w456] -> w395 mode=indexing
                      tunnel: w405 -> [w453]
                      tunnel: w404 -> [w455]
                      tunnel: w403 -> [w452]
                      tunnel: [w439] -> w399
                      tunnel: [w448] -> w398 mode=indexing
                      tunnel: [w446] -> w397 mode=indexing
                      tunnel: [w444] -> w396 mode=indexing
                      tunnel: "Temp Schedule" -> [w440]
                      tunnel: w393 -> [w438]
                      tunnel: w392 -> [w437]
                      tunnel: [w435] -> w391
                      tunnel: [w433] -> w390
                      tunnel: [w430] -> w389 mode=indexing
                      tunnel: [w426] -> w377
                      tunnel: [w425] -> w378
                      tunnel: w388 -> [w423]
                      tunnel: w387 -> [w422]
                      tunnel: [w420] -> w386 mode=indexing
                      shift-right: [w419] -> _
                      shift-left: 4.0 -> [w417]
                      tunnel: [w414] -> w385
                      tunnel: w383 -> [w413]
                      tunnel: w382 -> [w412]
                      tunnel: [w411] -> w381
                      tunnel: [w409] -> w380
                      tunnel: [w406] -> w379 mode=indexing
                      i -> [w439]
                      stop <- w432 stop-if-true
                      # "Loop will stop when button is pushed or in case of error."
                      n219 = flat-sequence {
                        tunnel: w455 -> [w492]
                        tunnel: w453 -> [w473]
                        tunnel: w452 -> [w519]
                        tunnel: [w520] -> w451
                        tunnel: [w506] -> w450
                        tunnel: [w472] -> w449
                        tunnel: [w480] -> w447
                        tunnel: [w481] -> w445
                        tunnel: [w486] -> w443
                        tunnel: [w505] -> w442
                        tunnel: w440 -> [w504]
                        tunnel: w439 -> [w502]
                        tunnel: w438 -> [w501]
                        tunnel: w437 -> [w500]
                        tunnel: [w499] -> w436
                        tunnel: [w498] -> w434
                        tunnel: [w467] -> w429
                        tunnel: [w489] -> w428
                        tunnel: [w488] -> w424
                        tunnel: w423 -> [w485]
                        tunnel: w422 -> [w484]
                        tunnel: [w477] -> w421
                        tunnel: [w477] -> w418
                        tunnel: w417 -> [w476]
                        tunnel: [w475] -> w416
                        tunnel: w413 -> [w462]
                        tunnel: w412 -> [w461]
                        tunnel: [w460] -> w410
                        tunnel: [w459] -> w408
                        tunnel: [w458] -> w407
                        tunnel: [w542] -> w454
                        tunnel: [w543] -> w456
                        tunnel: [w544] -> w457
                        tunnel: w451 -> [w544]
                        tunnel: w450 -> [w543]
                        tunnel: w449 -> [w542]
                        tunnel: [w540] -> w448
                        tunnel: w447 -> [w540]
                        tunnel: [w539] -> w446
                        tunnel: w445 -> [w539]
                        tunnel: [w538] -> w444
                        tunnel: w443 -> [w538]
                        tunnel: [w537] -> w435
                        tunnel: w436 -> [w537]
                        tunnel: [w536] -> w433
                        tunnel: w434 -> [w536]
                        tunnel: [w535] -> w430
                        tunnel: w429 -> [w535]
                        tunnel: [w534] -> w426
                        tunnel: w428 -> [w534]
                        tunnel: [w533] -> w425
                        tunnel: w424 -> [w533]
                        tunnel: w421 -> [w532]
                        tunnel: [w532] -> w420
                        tunnel: [w531] -> w419
                        tunnel: w418 -> [w531]
                        tunnel: [w530] -> w414
                        tunnel: w416 -> [w530]
                        tunnel: [w529] -> w411
                        tunnel: w410 -> [w529]
                        tunnel: [w528] -> w409
                        tunnel: w408 -> [w528]
                        tunnel: [w527] -> w406
                        tunnel: w407 -> [w527]
                        frame #0 {
                          # "Plot data on front panel"
                          # "Convert from V to T"
                          # "Filter"
                          # "Read Temp"
                          # "Read Temperature form Power Supply"
                          # "Set Current and measure Current and voltage."
                          # "Calculate Setpoint"
                          # "Create Timestamp"
                          # "PID Algorithm"
                          # "Alarms"
                          n220 = call-poly <userlib>:"OLRead.vi"("error in (no error)"=w461, "Task In"=w462) -> ("error out"=w459:errorcluster, "Data Value"=w463:dbl, "Task Out"=w460:refnum<k24>)  [unwired: 7 in]
                          n221 = call "Instrument I/O Assistant4"("Session In"=w485, "error in"=w484) -> ("Session Out"=w488:refnum<visa-resource-name>, "Temperature [C]"=w467:dbl, "error out"=w489:errorcluster)  [unwired: 23 in]
                          "Thermocouple Temperature [C]" <- w467
                          n222 = Equal?(x=w502, y=0.0) -> (x = y?=w487:bool)
                          n223 = call <vilib>:"PID Setpoint Profile.vi"("reinitialize? (F)"=w487, "setpoint profile"=w504) -> ("elapsed time (s)"=w506:dbl, "profile complete?"=w505:bool, "setpoint"=w486:dbl)  [unwired: 4 in, 1 out]
                          "Temperature Setpoint [C]" <- w486
                          n224 = Select(t=w476, s="Resistance?", f=w467) -> (s? t:f=w478:dbl)
                          n225 = call <vilib>:"Mean PtByPt.vi"("x"=w463, "sample length"=5 ("rank")) -> ("mean"=w466:dbl)  [unwired: 2 in, 1 out]
                          n226 = Multiply(x=1000.0, y=w466) -> (x*y=w458:dbl)
                          "Pyrometer Temperature [C]" <- w458
                          n227 = call-poly <vilib>:"PID Gain Schedule.vi"("PID gain schedule"="Gain Schedule", "gain scheduling value"=w478) -> ("PID gains out"=w483:T5)  [unwired: 2 in, 1 out]
                          n228 = call-poly <vilib>:"PID.vi"("reinitialize? (F)"=w487, "output range"=cluster{"output high":dbl, "output low":dbl} {"output high"=1000.0, "output low"=0.0}, "PID gains"=w483, "process variable"=w467, "setpoint"=w486) -> ("output"=w469:dbl)  [unwired: 5 in, 1 out]
                          n229 = Subtract(x=w492, y=0.1) -> (x-y=w509:dbl)
                          n230 = Add(x=0.1, y=w492) -> (x+y=w497:dbl)
                          n231 = Add(x=0.1, y=w473) -> (x+y=w493:dbl)
                          n232 = case shown="True" "OutputPower?" {
                            tunnel: [errorcluster {"status"=FALSE, "code"=0, "source"=""} ("error IO") w526] -> w475
                            tunnel: w469 -> [w522 w525]
                            tunnel: [w522 w524] -> w468
                            tunnel: w467 -> [_ w523]
                            frame #0 {
                            }
                            frame #1 {
                              n233 = script code="if T < 530\n    R = 7.470;\nelseif T < 810\n    R = -.01371*T+15.01;\nelse\n    R = 3.905;\nend\n\nI = P/(R^2);"("P"=w525, "T"=w523) -> ("??"=w526:errorcluster, "I"=w524:dbl)  [unwired: 1 in]
                            }
                          }
                          n234 = Subtract(x=w473, y=0.1 ("x")) -> (x-y=w491:dbl)
                          n235 = Greater?(x=w467, y=w519) -> (0:→"Over Temperature":bool)
                          n236 = In Range and Coerce(upper limit=w473, x=w468, lower limit=0.0) -> (coerced(x)=w472:dbl)  [unwired: 1 out]
                          "Current Setpoint [A]" <- w472
                          n237 = call "Instrument I/O Assistant2"("Session In"=w501, "Input Current [A]"=w472, "error in"=w500) -> ("Session Out"=w499:refnum<visa-resource-name>, "Measured Current [A]"=w480:dbl, "Measured Voltage [V]"=w481:dbl, "error out"=w498:errorcluster)  [unwired: 21 in]
                          "Measured Voltage [V]" <- w481
                          "Measured Current [A]" <- w480
                          n238 = Bundle(w458, "Temperature [C]"=w467, "setpoint"=w486, "Measured Current [A]"=w480) -> (→"Temperature and Current v. Time":T2)  [unwired: 1 in]
                          n239 = Greater?(x=w481, y=w492) -> (0:→"Over Voltage":bool)
                          n240 = Greater?(x=w480, y=w473) -> (0:→"Over Current":bool)
                          n241 = In Range and Coerce(upper limit=w497, x=w481, lower limit=w509) -> (In Range?=→"Maximum Voltage":bool)  [unwired: 1 out]
                          n242 = In Range and Coerce(upper limit=w493, x=w480, lower limit=w491) -> (In Range?=→"Maximum Current":bool)  [unwired: 1 out]
                          n243 = Get Date/Time String(date format (0)=enum16{"short", "long", "abbreviated"}."short", want seconds? (F)=TRUE) -> (date string=w516:string, time string=w515:string)  [unwired: 1 in]
                          n244 = call <vilib>:"Space Constant.vi"() -> ("String"=w514:string)
                          n245 = Divide(x=w481, y=w480) -> (x/y=w477:dbl)
                          "Measured Resistance [ohms]" <- w477
                          n246 = Concatenate Strings(w516, w514, w515) -> (w520:string)
                        }
                        frame #1 {
                          # "Wait for next 500 ms increment."
                          n247 = Wait Until Next ms Multiple(millisecond multiple=u32 500) -> ()  [unwired: 1 out]
                        }
                      }
                      n248 = Unbundle By Name(w414) -> ("status"=w415:bool)
                      n249 = Unbundle By Name(w433) -> ("status"=w431:bool)
                      n250 = Unbundle By Name(w426) -> ("status"=w427:bool)
                      n251 = Compound Arithmetic op=OR(w415, w427, w431, "Stop Heating", w442) -> (w432:bool)
                      "Stop Running" <- w432
                    }
                    "Current Setpoint" <- w402
                    "Time" <- w395
                    "Date" <- w401
                    "Pyrometer Temperature" <- w379
                    "Temperature Setpoint" <- w396
                    "Current" <- w398
                    "Voltage" <- w397
                    "Thermocouple Temperature" <- w389
                    "Resistance" <- w386
                    n252 = Increment(x=w399) -> (x+1=→"Data Points":i32)
                    n253 = call <vilib>:"Simple Error Handler.vi"("error in (no error)"=w385) -> ()  [unwired: 4 in, 5 out]
                  }
                }
                n254 = call "Instrument I/O Assistant3"("Session In"=w358, "error in"=w357) -> ("Session Out"=w355:refnum<visa-resource-name>, "error out"=w356:errorcluster)  [unwired: 24 in]
                n255 = VISA Close(VISA resource name=w336, error in (no error)=w335) -> (error out=w337:errorcluster)
                n256 = call <userlib>:"OLCloseTask.vi"("Error in"=w342, "Task In"=w341) -> ("Error Out"=w340:errorcluster)  [unwired: 9 in]
                n257 = call <vilib>:"Simple Error Handler.vi"("error in (no error)"=w337) -> ()  [unwired: 4 in, 5 out]
                n258 = VISA Close(VISA resource name=w355, error in (no error)=w356) -> (error out=w354:errorcluster)
                n259 = call <vilib>:"Simple Error Handler.vi"("error in (no error)"=w340) -> ()  [unwired: 4 in, 5 out]
                n260 = call <vilib>:"Simple Error Handler.vi"("error in (no error)"=w354) -> ()  [unwired: 4 in, 5 out]
              }
              frame #3 {
                w553 = FALSE
                # "Change greyed out inputs and outputs"
                n261 = property on="Current Setpoint [A]" class="DigNum (strict)"("Disabled"=u8 2) -> ()  [unwired: 2 in, 2 out]
                n262 = property on="Measured Resistance [ohms]" class="DigNum (strict)"("DisabledEnum"=2) -> ()  [unwired: 2 in, 2 out]
                n263 = property on="Thermocouple Temperature [C]" class="DigNum (strict)"("DisabledEnum"=2) -> ()  [unwired: 2 in, 2 out]
                n264 = property on="Measured Current [A]" class="DigNum (strict)"("DisabledEnum"=2) -> ()  [unwired: 2 in, 2 out]
                n265 = property on="Measured Voltage [V]" class="DigNum (strict)"("DisabledEnum"=2) -> ()  [unwired: 2 in, 2 out]
                n266 = property on="Current Limit [A]" class="DigNum (strict)"("Disabled"=0) -> ()  [unwired: 2 in, 2 out]
                n267 = property on="Temperature Limit [C]" class="DigNum (strict)"("Disabled"=0) -> ()  [unwired: 2 in, 2 out]
                n268 = property on="End Program" class="Bool"("Disabled"=0) -> ()  [unwired: 2 in, 2 out]
                n269 = property on="Voltage Limit [V]" class="DigNum (strict)"("Disabled"=0) -> ()  [unwired: 2 in, 2 out]
                n270 = property on="Set Temperature" class="Bool"("DisabledEnum"=0) -> ()  [unwired: 2 in, 2 out]
                n271 = property on="Gain Schedule" class="Bool"("DisabledEnum"=0) -> ()  [unwired: 2 in, 2 out]
                n272 = property on="Reset" class="Bool"("Disabled"=0) -> ()  [unwired: 2 in, 2 out]
                n273 = property on="Stop Heating" class="Bool (strict)"("Disabled"=2) -> ()  [unwired: 2 in, 2 out]
                n274 = property on="Pyrometer Temperature [C]" class="DigNum (strict)"("DisabledEnum"=u8 2 ("Disabled")) -> ()  [unwired: 2 in, 2 out]
                n275 = property on="Save Data" class="Bool (strict)"("Disabled"=u8 0) -> ()  [unwired: 2 in, 2 out]
                n276 = property on="Maximum Current" class="Bool (strict)"("Value"=w553) -> ()  [unwired: 2 in, 2 out]
                n277 = property on="Over Voltage" class="Bool (strict)"("Value"=w553) -> ()  [unwired: 2 in, 2 out]
                n278 = property on="Over Temperature" class="Bool (strict)"("Value"=w553) -> ()  [unwired: 2 in, 2 out]
                n279 = property on="Maximum Voltage" class="Bool (strict)"("Value"=w553) -> ()  [unwired: 2 in, 2 out]
                n280 = property on="Temperature Setpoint [C]" class="DigNum (strict)"("DisabledEnum"=2) -> ()  [unwired: 2 in, 2 out]
                n281 = property on="Over Current" class="Bool (strict)"("Value"=w553) -> ()  [unwired: 2 in, 2 out]
                n282 = local write "Stop Heating"(w553) -> ()
              }
            }
          }
        }
      }
    }
  }
